vi "Demo.vi"() -> ()   [LabVIEW 2018]
uses:
  Demo_Commands.ctl
panel:
  in  "Scanner brake":bool
  out "new data":bool
  in  "Analog out GAIN":u16(ring) items=["1", "10", "100"]
  in  "Reset":bool
  in  "FIND":bool
  in  "DAF":dbl format="%#_6f"
  out "info string":string="to start measurement press record"
  in  "Scanner Offset":sgl min=-756 max=756
  in  "Scanner Amplitude":sgl=1.0 min=0 max=56
  out "connected":bool=TRUE
  in  "Scanner Frequency":dbl min=0.1 max=25.0
  in  "Sample Frequency":dbl min=0.4 max=50.0
  in  "exit":bool
  in  "Resource":i32(listbox)
  in  "Power Amp":bool
  out "Signalverlaufsgraph":dbl[](graph)
  out "Amplitude":dbl
  in  "Scan":bool
  out "VISA SD":refnum<visa-resource-name>
  out "VISA Error Out":errorcluster
  in  "Connect":bool
  out "ExtTrigFreq (Hz)":dbl format="%.3f"
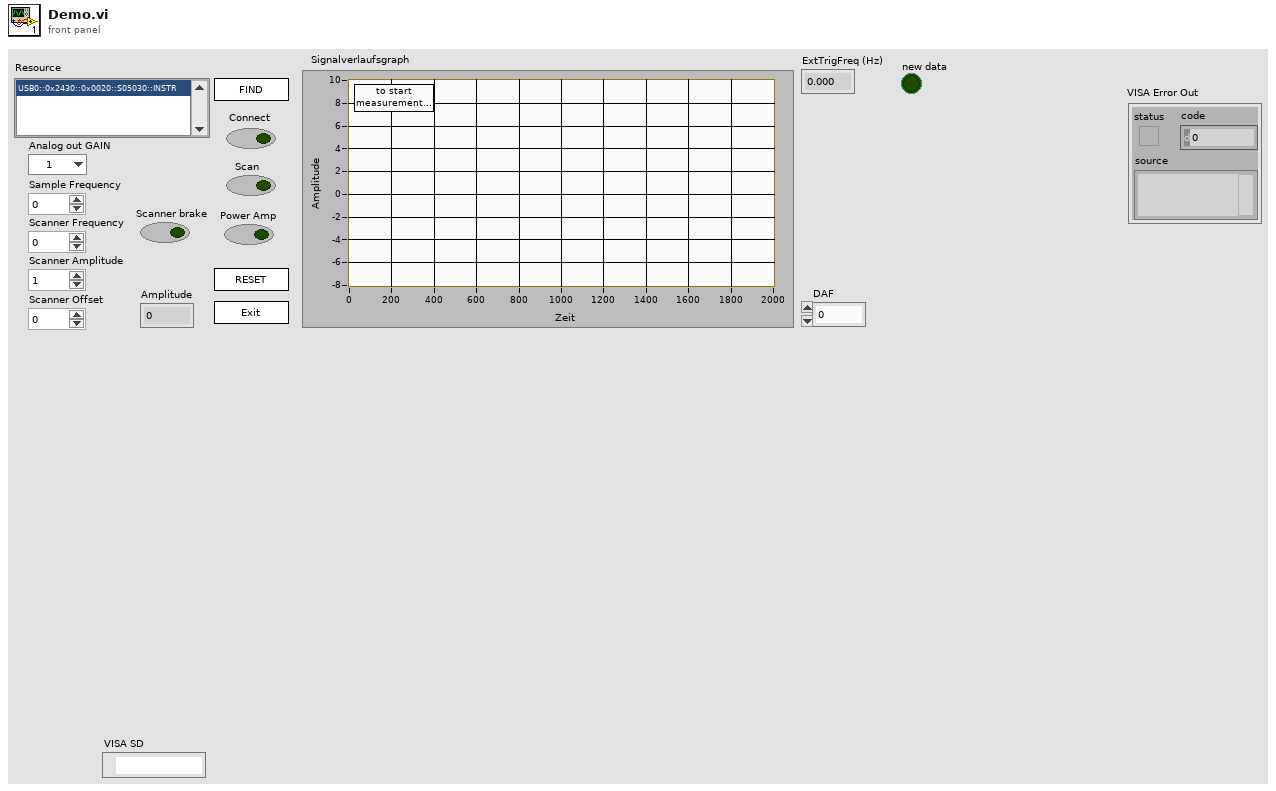
[diagram p1: front panel]
types:
  T1 = typedef "Demo_Commands.ctl" = enum16{"find", "connect", "exit", "get data", "sample frequency", "scan frequency", "power amp", "scanner brake", "reset", "monitor gain", "scan amplitude", "scan offset"}
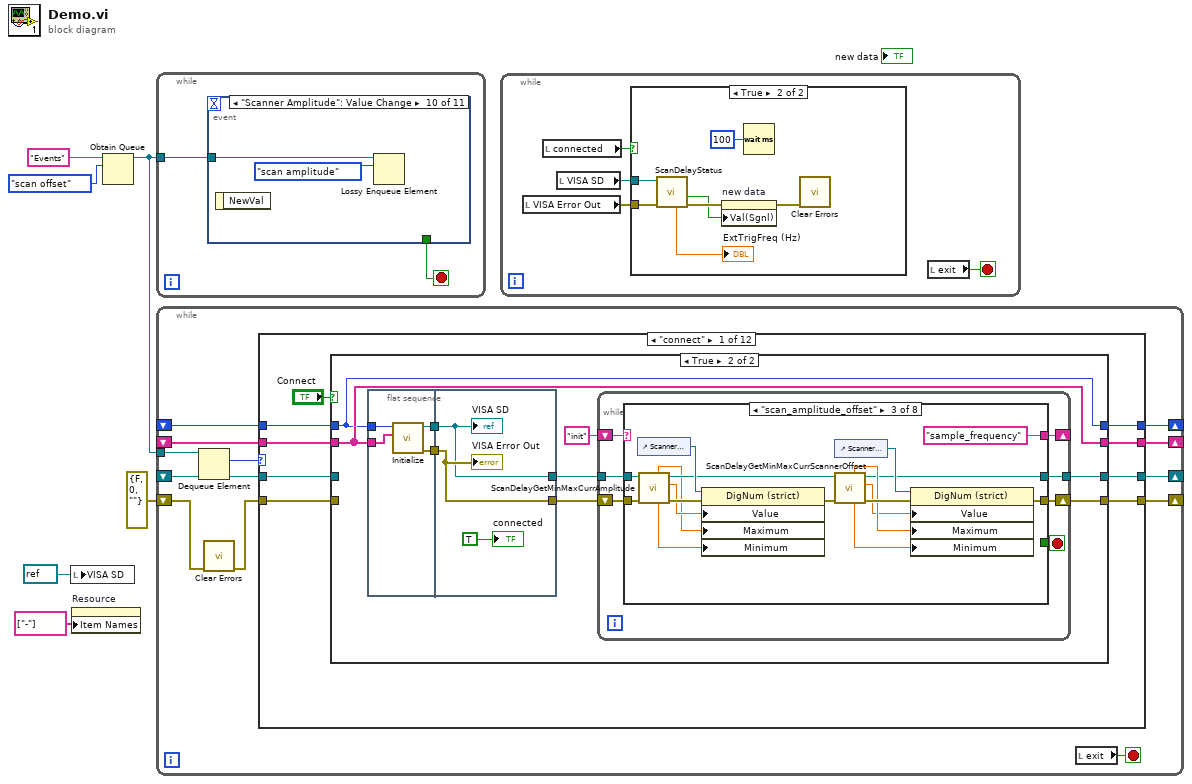
[diagram p0: block diagram]
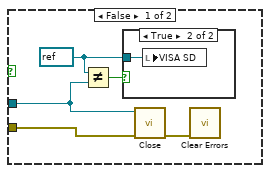
[diagram p2: hidden frame]
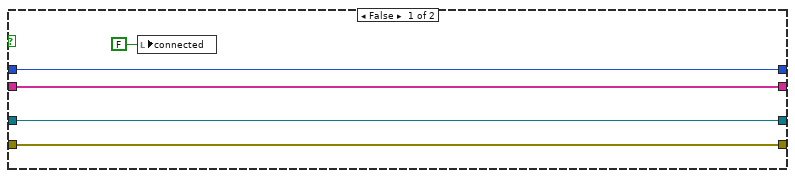
[diagram p4: hidden frame]
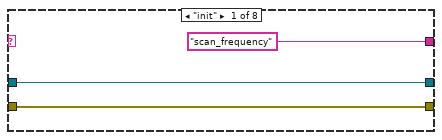
[diagram p5: hidden frame]
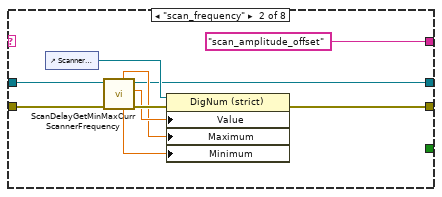
[diagram p6: hidden frame]
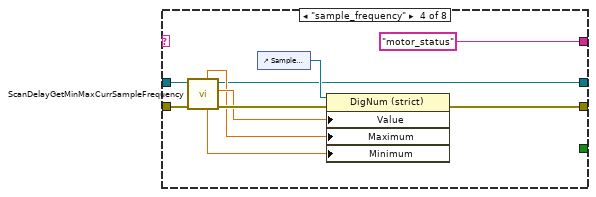
[diagram p7: hidden frame]
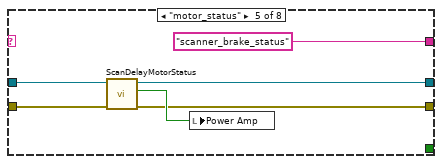
[diagram p8: hidden frame]
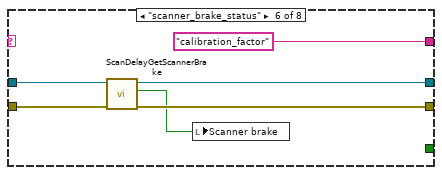
[diagram p9: hidden frame]
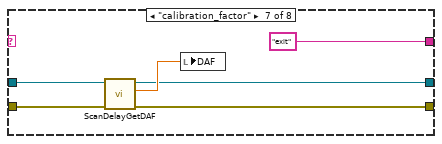
[diagram p10: hidden frame]
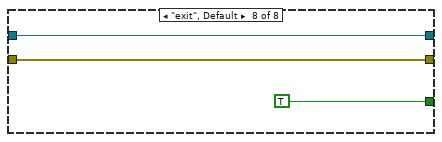
[diagram p11: hidden frame]
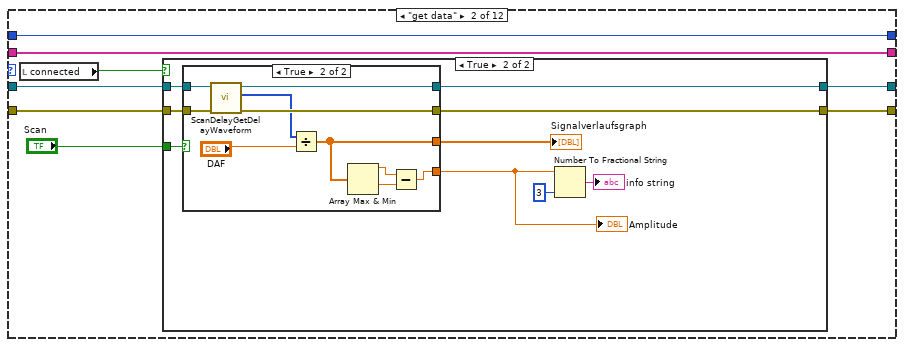
[diagram p12: hidden frame]
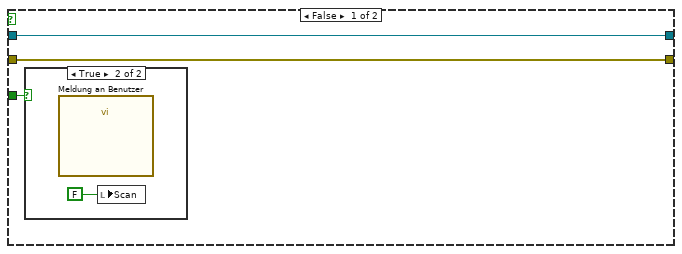
[diagram p13: hidden frame]
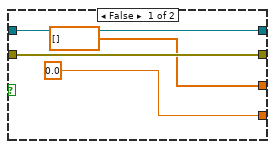
[diagram p15: hidden frame]
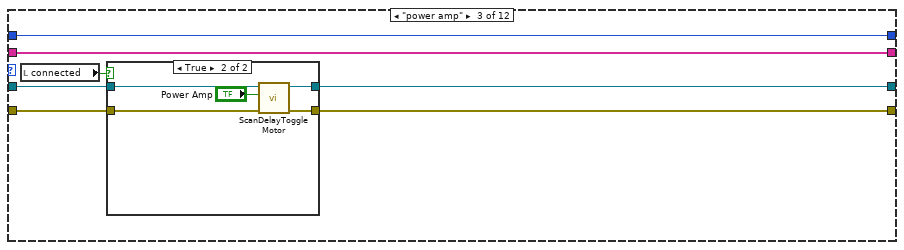
[diagram p16: hidden frame]
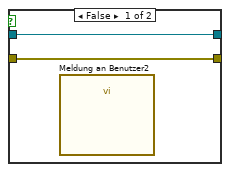
[diagram p17: hidden frame]
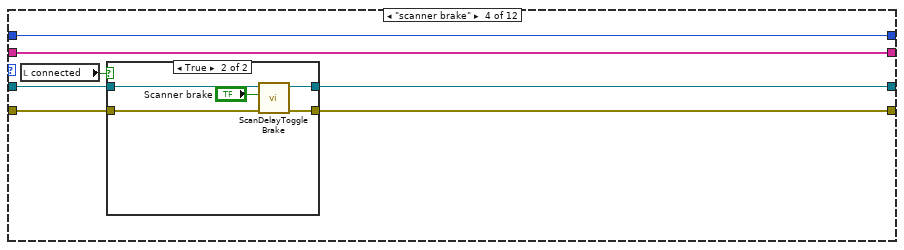
[diagram p18: hidden frame]
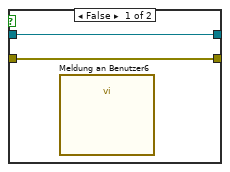
[diagram p19: hidden frame]
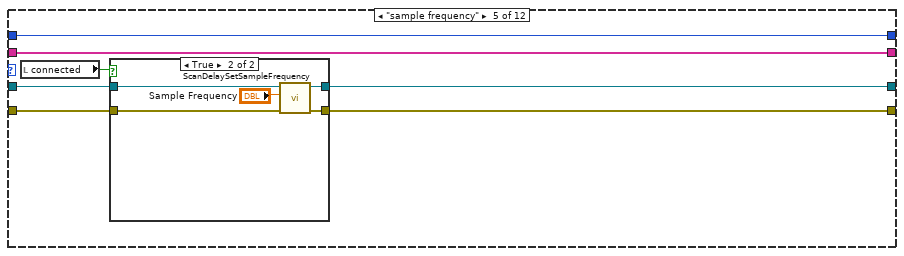
[diagram p20: hidden frame]
diagram:
  n1 = local write "VISA SD"(refnum<visa-resource-name> "0" ("VISA SD")) -> ()
  n2 = property on="Resource" class="LstBox (strict)"("Item Names"=string[] ["-"]) -> ()  [unwired: 2 in, 2 out]
  n3 = Obtain Queue(name (unnamed)="Events" ("Name (unbenannt)"), element data type=Demo_Commands."scan offset" ("element")) -> (queue out=w5:refnum<queue>)  [unwired: 3 in, 2 out]
  n4 = while {
    tunnel: w5 -> [w8]
    stop <- w7 stop-if-true
    n5 = event shown="[9] \"Scanner Amplitude\": Value Change" {
      selector: _ -> [_ _ _ _ _ _ _ _ _ _ _]
      dyn-events: _ -> [_ _ _ _ _ _ _ _ _ _ _]
      timeout: _ -> [_ _ _ _ _ _ _ _ _ _ _]
      tunnel: w8 -> [w10 w12 w15 w17 w19 w21 w23 w25 w27 w29 w31]
      tunnel: [_ _ "exit" _ _ _ _ _ _ _ _] -> w7
      event "FIND": Value Change {
        n6 = event-data() -> ()  [unwired: 1 in, 1 out]
        n7 = Lossy Enqueue Element(queue=w10, element=Demo_Commands."find" ("Befehlssatz")) -> ()  [unwired: 1 in, 4 out]
      }
      event "Connect": Value Change {
        n8 = event-data() -> ()  [unwired: 1 in, 1 out]
        n9 = Lossy Enqueue Element(queue=w12, element=Demo_Commands."connect" ("Befehlssatz")) -> ()  [unwired: 1 in, 4 out]
      }
      event "exit": Value Change {
        n10 = event-data() -> ()  [unwired: 1 in, 1 out]
        n11 = Lossy Enqueue Element(queue=w15, element=Demo_Commands."exit" ("Befehlssatz")) -> ()  [unwired: 1 in, 4 out]
      }
      event "new data", "Scan": Value Change {
        n12 = event-data() -> ()  [unwired: 1 in, 1 out]
        n13 = Lossy Enqueue Element(queue=w17, element=Demo_Commands."get data" ("Befehlssatz")) -> ()  [unwired: 1 in, 4 out]
      }
      event "Reset": Value Change {
        n14 = event-data() -> ()  [unwired: 1 in, 1 out]
        n15 = Lossy Enqueue Element(queue=w19, element=Demo_Commands."reset" ("Befehlssatz")) -> ()  [unwired: 1 in, 4 out]
      }
      event "Sample Frequency": Value Change {
        n16 = event-data() -> ()  [unwired: 1 in, 1 out]
        n17 = Lossy Enqueue Element(queue=w21, element=Demo_Commands."sample frequency" ("Befehlssatz")) -> ()  [unwired: 1 in, 4 out]
      }
      event "Scanner Frequency": Value Change {
        n18 = event-data() -> ()  [unwired: 1 in, 1 out]
        n19 = Lossy Enqueue Element(queue=w23, element=Demo_Commands."scan frequency" ("Befehlssatz")) -> ()  [unwired: 1 in, 4 out]
      }
      event "Analog out GAIN": Value Change {
        n20 = event-data() -> ()  [unwired: 1 in, 1 out]
        n21 = Lossy Enqueue Element(queue=w25, element=Demo_Commands."monitor gain" ("Befehlssatz")) -> ()  [unwired: 1 in, 4 out]
      }
      event "Power Amp": Value Change {
        n22 = event-data() -> ()  [unwired: 1 in, 1 out]
        n23 = Lossy Enqueue Element(queue=w27, element=Demo_Commands."power amp" ("Befehlssatz")) -> ()  [unwired: 1 in, 4 out]
      }
      event "Scanner Amplitude": Value Change {
        n24 = event-data() -> ()  [unwired: 1 in, 1 out]
        n25 = Lossy Enqueue Element(queue=w29, element=Demo_Commands."scan amplitude") -> ()  [unwired: 1 in, 4 out]
      }
      event "Scanner Offset": Value Change {
        n26 = event-data() -> ()  [unwired: 1 in, 1 out]
        n27 = Lossy Enqueue Element(queue=w31, element=Demo_Commands."scan offset") -> ()  [unwired: 1 in, 4 out]
      }
    }
  }
  n28 = while {
    tunnel: w5 -> [w42]
    shift-right: [w41] -> _
    shift-left: _ -> [w36]
    shift-right: [w40] -> _
    shift-left: _ -> [w39]
    shift-right: [w38] -> _
    shift-left: _ -> [w34]
    shift-right: [w37] -> _
    shift-left: errorcluster {"status"=FALSE, "code"=0, "source"=""} ("error out") -> [w33]
    stop <- w35 stop-if-true
    n29 = Dequeue Element(queue=w42) -> (element=w43:T1)  [unwired: 2 in, 3 out]
    n30 = call <vilib>:"Clear Errors.vi"("error in (no error)"=w33) -> ("error out"=w32:errorcluster)  [unwired: 5 in, 1 out]
    n31 = case shown="\"connect\"" w43 {
      tunnel: [w44 w146 w177 w191 w205 w219 w232 "Resource" w243 w260 w275 w289] -> w41
      tunnel: [w45 w147 w178 w192 w206 w220 w235 w239 w244 w259 w274 w288] -> w40
      tunnel: w39 -> [w52 w147 w178 w192 w206 w220 w235 _ w244 w259 w274 w288]
      tunnel: [w50 w148 w180 w194 w208 w222 w233 refnum<visa-resource-name> refnum ("VISA resource name out") w246 w256 w272 w286] -> w38
      tunnel: [w51 w145 w179 w193 w207 w221 w234 w238 w245 w255 w273 w285] -> w37
      tunnel: w36 -> [w49 w146 w177 w191 w205 w219 w232 _ w243 w260 w275 w289]
      tunnel: w34 -> [w47 w144 w181 w195 w209 w223 w233 _ w247 w258 w271 w287]
      tunnel: w32 -> [w46 w143 w182 w196 w210 w224 w234 w236 w248 w257 w270 w284]
      frame "connect" {
        n32 = case shown="True" "Connect" {
          tunnel: w52 -> [w57 w66]
          tunnel: [w53 w62] -> w51
          tunnel: [w54 w61] -> w50
          tunnel: w49 -> [w56 w65]
          tunnel: w47 -> [w54 _]
          tunnel: w46 -> [w53 _]
          tunnel: [w57 w66] -> w45
          tunnel: [w56 w65] -> w44
          frame False {
            n33 = local write "connected"(FALSE ("connected")) -> ()
          }
          frame True {
            n34 = flat-sequence {
              tunnel: w66 -> [w136]
              tunnel: w65 -> [w137]
              tunnel: [w135] -> w59
              tunnel: [w134] -> w58
              tunnel: [w139] -> w63
              tunnel: [w140] -> w64
              tunnel: w59 -> [w140]
              tunnel: w58 -> [w139]
              frame #0 {
                n35 = call "Initialize.vi"("resource array"=w136, "Resource"=w137) -> ("VISA Error Out"=w135:errorcluster, "VISA  name out"=w134:refnum<visa-resource-name>)  [unwired: 7 in, 1 out]
              }
              frame #1 {
                "VISA Error Out" <- w140
                "VISA SD" <- w139
                "connected" <- TRUE
              }
            }
            n36 = while {
              tunnel: w63 -> [w72]
              shift-right: [w71] -> w62
              shift-left: w64 -> [w73]
              tunnel: [w70] -> w61
              shift-right: [w68] -> _
              shift-left: "init" -> [w69]
              stop <- w67 stop-if-true
              n37 = case shown="\"scan_amplitude_offset\"" w69 {
                tunnel: w73 -> [w75 w85 w99 w111 w116 w123 w127 w133]
                tunnel: w72 -> [w74 w84 w98 w110 w115 w122 w126 w132]
                tunnel: [w75 w86 w102 w105 w114 w121 w128 w133] -> w71
                tunnel: [w74 w78 w88 w104 w113 w120 w125 w132] -> w70
                tunnel: ["scan_frequency" "scan_amplitude_offset" "sample_frequency" "motor_status" "scanner_brake_status" "calibration_factor" "exit" _] -> w68
                tunnel: [_ _ _ _ _ _ _ TRUE] -> w67
                frame "init" {
                }
                frame "scan_frequency" {
                  n38 = control-ref of="Scanner Frequency"() -> (w83:refnum<vi>)
                  n39 = call "ScanDelayGetMinMaxCurrScannerFrequency.vi"("error in (no error)"=w85, "VISA resource name in"=w84) -> ("error out"=w82:errorcluster, "value"=w81:dbl, "VISA resource name out"=w78:refnum<visa-resource-name>, "min"=w79:dbl, "max"=w80:dbl)  [unwired: 5 in]
                  n40 = property class="DigNum (strict)"(reference=w83, error in=w82, "Value"=w81, "Maximum"=w80, "Minimum"=w79) -> (error out=w86:errorcluster)  [unwired: 1 out]
                }
                frame "scan_amplitude_offset" {
                  n41 = control-ref of="Scanner Amplitude"() -> (w100:refnum<vi>)
                  n42 = call "ScanDelayGetMinMaxCurrAmplitude.vi"("error in (no error)"=w99, "VISA resource name in"=w98) -> ("error out"=w97:errorcluster, "value"=w95:dbl, "VISA resource name out"=w89:refnum<visa-resource-name>, "min"=w96:dbl, "max"=w87:dbl)  [unwired: 5 in]
                  n43 = property class="DigNum (strict)"(reference=w100, error in=w97, "Value"=w95, "Maximum"=w87, "Minimum"=w96) -> (error out=w102:errorcluster)  [unwired: 1 out]
                  n44 = control-ref of="Scanner Offset"() -> (w90:refnum<vi>)
                  n45 = call "ScanDelayGetMinMaxCurrScannerOffset.vi"("VISA resource name in"=w89) -> ("error out"=w92:errorcluster, "value"=w91:dbl, "VISA resource name out"=w88:refnum<visa-resource-name>, "min"=w94:dbl, "max"=w93:dbl)  [unwired: 6 in]
                  n46 = property class="DigNum (strict)"(reference=w90, error in=w92, "Value"=w91, "Maximum"=w93, "Minimum"=w94) -> ()  [unwired: 2 out]
                }
                frame "sample_frequency" {
                  n47 = call "ScanDelayGetMinMaxCurrSampleFrequency.vi"("error in (no error)"=w111, "VISA resource name in"=w110) -> ("error out"=w109:errorcluster, "value"=w108:dbl, "VISA resource name out"=w104:refnum<visa-resource-name>, "min"=w106:dbl, "max"=w107:dbl)  [unwired: 5 in]
                  n48 = control-ref of="Sample Frequency"() -> (w112:refnum<vi>)
                  n49 = property class="DigNum (strict)"(reference=w112, error in=w109, "Value"=w108, "Maximum"=w107, "Minimum"=w106) -> (error out=w105:errorcluster)  [unwired: 1 out]
                }
                frame "motor_status" {
                  n50 = call "ScanDelayMotorStatus.vi"("error in (no error)"=w116, "VISA resource name in"=w115) -> ("error out"=w114:errorcluster, "value"=w117:bool, "VISA resource name out"=w113:refnum<visa-resource-name>)  [unwired: 7 in]
                  n51 = local write "Power Amp"(w117) -> ()
                }
                frame "scanner_brake_status" {
                  n52 = call "ScanDelayGetScannerBrake.vi"("error in (no error)"=w123, "VISA resource name in"=w122) -> ("error out"=w121:errorcluster, "value"=w119:bool, "VISA resource name out"=w120:refnum<visa-resource-name>)  [unwired: 7 in]
                  n53 = local write "Scanner brake"(w119) -> ()
                }
                frame "calibration_factor" {
                  n54 = call "ScanDelayGetDAF.vi"("error in (no error)"=w127, "VISA resource name in"=w126) -> ("error out"=w128:errorcluster, "value"=w129:dbl, "VISA resource name out"=w125:refnum<visa-resource-name>)  [unwired: 7 in]
                  n55 = local write "DAF"(w129) -> ()
                }
                frame "exit", Default {
                }
              }
            }
          }
        }
      }
      frame "get data" {
        n56 = local read "connected"() -> (w142:bool)
        n57 = case shown="True" w142 {
          tunnel: [w151 w161] -> w148
          tunnel: [w150 w160] -> w145
          tunnel: w144 -> [w151 w159]
          tunnel: w143 -> [w150 w158]
          tunnel: "Scan" -> [w149 w157]
          frame False {
            n58 = case shown="True" w149 {
              frame False {
              }
              frame True {
                n59 = call "Meldung an Benutzer"() -> ()  [unwired: 10 in, 2 out]
                n60 = local write "Scan"(FALSE ("Scann")) -> ()
              }
            }
          }
          frame True {
            n61 = case shown="True" w157 {
              tunnel: w158 -> [w164 w175]
              tunnel: w159 -> [w165 w174]
              tunnel: [w165 w173] -> w161
              tunnel: [w164 w172] -> w160
              tunnel: [dbl[] [] ("PSD Waveform") w169] -> w155
              tunnel: [0.0 ("Amplitude") w166] -> w154
              frame False {
              }
              frame True {
                n62 = call "ScanDelayGetDelayWaveform.vi"("error in (no error)"=w175, "VISA resource name in"=w174) -> ("error out"=w172:errorcluster, "values"=w170:i16[], "VISA resource name out"=w173:refnum<visa-resource-name>)  [unwired: 7 in]
                n63 = Divide(x=w170, y="DAF") -> (x/y=w169:dbl[])
                n64 = Array Max & Min(array=w169) -> (max value=w168:dbl, min value=w167:dbl)  [unwired: 2 out]
                n65 = Subtract(x=w168, y=w167) -> (x-y=w166:dbl)
              }
            }
            "Signalverlaufsgraph" <- w155
            "Amplitude" <- w154
            n66 = Number To Fractional String(number=w154, precision (6)=i16 3) -> (F-format string=→"info string":string)  [unwired: 2 in]
          }
        }
      }
      frame "power amp" {
        n67 = local read "connected"() -> (w176:bool)
        n68 = case shown="True" w176 {
          tunnel: w182 -> [w183 w189]
          tunnel: w181 -> [w184 w188]
          tunnel: [w184 w186] -> w180
          tunnel: [w183 w185] -> w179
          frame False {
            n69 = call "Meldung an Benutzer2"() -> ()  [unwired: 10 in, 2 out]
          }
          frame True {
            n70 = call "ScanDelayToggleMotor.vi"("error in (no error)"=w189, "value"="Power Amp", "VISA resource name in"=w188) -> ("error out"=w185:errorcluster, "VISA resource name out"=w186:refnum<visa-resource-name>)  [unwired: 7 in]
          }
        }
      }
      frame "scanner brake" {
        n71 = local read "connected"() -> (w190:bool)
        n72 = case shown="True" w190 {
          tunnel: w196 -> [w197 w203]
          tunnel: w195 -> [w198 w202]
          tunnel: [w198 w201] -> w194
          tunnel: [w197 w200] -> w193
          frame False {
            n73 = call "Meldung an Benutzer6"() -> ()  [unwired: 10 in, 2 out]
          }
          frame True {
            n74 = call "ScanDelayToggleBrake.vi"("error in (no error)"=w203, "value"="Scanner brake", "VISA resource name in"=w202) -> ("error out"=w200:errorcluster, "VISA resource name out"=w201:refnum<visa-resource-name>)  [unwired: 7 in]
          }
        }
      }
      frame "sample frequency" {
        n75 = local read "connected"() -> (w204:bool)
        n76 = case shown="True" w204 {
          tunnel: w210 -> [w211 w217]
          tunnel: w209 -> [w212 w216]
          tunnel: [w212 w215] -> w208
          tunnel: [w211 w214] -> w207
          frame False {
            n77 = call "Meldung an Benutzer3"() -> ()  [unwired: 10 in, 2 out]
          }
          frame True {
            n78 = call "ScanDelaySetSampleFrequency.vi"("error in (no error)"=w217, "value"="Sample Frequency", "VISA resource name in"=w216) -> ("error out"=w214:errorcluster, "VISA resource name out"=w215:refnum<visa-resource-name>)  [unwired: 7 in]
          }
        }
      }
      frame "scan frequency" {
        n79 = local read "connected"() -> (w218:bool)
        n80 = case shown="True" w218 {
          tunnel: w224 -> [w225 w231]
          tunnel: w223 -> [w226 w230]
          tunnel: [w226 w229] -> w222
          tunnel: [w225 w228] -> w221
          frame False {
            n81 = call "Meldung an Benutzer4"() -> ()  [unwired: 10 in, 2 out]
          }
          frame True {
            n82 = call "ScanDelaySetScannerFrequency.vi"("error in (no error)"=w231, "value"="Scanner Frequency", "VISA resource name in"=w230) -> ("error out"=w228:errorcluster, "VISA resource name out"=w229:refnum<visa-resource-name>)  [unwired: 7 in]
          }
        }
      }
      frame "exit" {
      }
      frame "find" {
        n83 = call "FindResource.vi"("error in (no error)"=w236) -> ("error out"=w238:errorcluster, "resource array"=w241:string[])  [unwired: 8 in, 1 out]
        n84 = property on="Resource" class="LstBox (strict)"("Item Names"=w241) -> ("Item Names"=w239:string[])  [unwired: 2 in, 2 out]
      }
      frame "reset" {
        n85 = local read "connected"() -> (w242:bool)
        n86 = case shown="True" w242 {
          tunnel: w248 -> [w249 w254]
          tunnel: w247 -> [w250 w253]
          tunnel: [w250 w252] -> w246
          tunnel: [w249 w251] -> w245
          frame False {
            n87 = call "Meldung an Benutzer5"() -> ()  [unwired: 10 in, 2 out]
          }
          frame True {
            n88 = call "Reset.vi"("error in (no error)"=w254, "VISA resource name"=w253) -> ("error out"=w251:errorcluster, "VISA resource name out"=w252:refnum<visa-resource-name>)  [unwired: 8 in]
          }
        }
      }
      frame "monitor gain" {
        n89 = local read "connected"() -> (w261:bool)
        n90 = case shown="True" w261 {
          tunnel: w258 -> [w263 w268]
          tunnel: w257 -> [w262 w267]
          tunnel: [w263 w266] -> w256
          tunnel: [w262 w265] -> w255
          frame False {
          }
          frame True {
            n91 = call "ScanDelaySetMonitorGain.vi"("error in (no error)"=w267, "wait"="Analog out GAIN", "VISA resource name in"=w268) -> ("error out"=w265:errorcluster, "VISA resource name out"=w266:refnum<visa-resource-name>)  [unwired: 7 in]
          }
        }
      }
      frame "scan amplitude" {
        n92 = local read "connected"() -> (w269:bool)
        n93 = case shown="True" w269 {
          tunnel: [w276 w282] -> w273
          tunnel: [w277 w281] -> w272
          tunnel: w271 -> [w277 w280]
          tunnel: w270 -> [w276 w279]
          frame False {
          }
          frame True {
            n94 = call "ScanDelaySetAmplitude.vi"("error in (no error)"=w279, "value"="Scanner Amplitude", "VISA resource name in"=w280) -> ("error out"=w282:errorcluster, "VISA resource name out"=w281:refnum<visa-resource-name>)  [unwired: 7 in]
          }
        }
      }
      frame "scan offset" {
        n95 = local read "connected"() -> (w283:bool)
        n96 = case shown="True" w283 {
          tunnel: w287 -> [w291 w296]
          tunnel: [w291 w295] -> w286
          tunnel: [w290 w294] -> w285
          tunnel: w284 -> [w290 w293]
          frame False {
          }
          frame True {
            n97 = call "ScanDelaySetScannerOffset.vi"("error in (no error)"=w293, "value"="Scanner Offset", "VISA resource name in"=w296) -> ("error out"=w294:errorcluster, "VISA resource name out"=w295:refnum<visa-resource-name>)  [unwired: 7 in]
          }
        }
      }
    }
    n98 = local read "exit"() -> (w35:bool)
  }
  n99 = while {
    stop <- w298 stop-if-true
    n100 = local read "VISA Error Out"() -> (w299:errorcluster)
    n101 = local read "connected"() -> (w297:bool)
    n102 = local read "VISA SD"() -> (w300:refnum<visa-resource-name>)
    n103 = case shown="True" w297 {
      tunnel: w300 -> [w303 w313]
      tunnel: w299 -> [w305 w312]
      frame False {
        w302 = refnum<visa-resource-name> "0" ("VISA SD")
        n104 = Not Equal?(x=w302, y=w303) -> (x != y?=w301:bool)
        n105 = case shown="True" w301 {
          tunnel: w302 -> [_ w306]
          frame False {
          }
          frame True {
            n106 = local write "VISA SD"(w306) -> ()
          }
        }
        n107 = call "Close.vi"("error in (no error)"=w305, "VISA resource name"=w303) -> ("error out"=w304:errorcluster)  [unwired: 9 in]
        n108 = call <vilib>:"Clear Errors.vi"("error in (no error)"=w304) -> ()  [unwired: 5 in, 2 out]
      }
      frame True {
        n109 = call "ScanDelayStatus.vi"("error in"=w312, "VISA APE resource"=w313) -> ("error out"=w310:errorcluster, "new data"=w309:bool, "External trigger frequency (Hz)"=→"ExtTrigFreq (Hz)":dbl)  [unwired: 4 in, 3 out]
        n110 = property on="new data" class="Bool (strict)"(error in=w310, "Val(Sgnl)"=w309) -> (error out=w307:errorcluster)  [unwired: 1 in, 1 out]
        n111 = Wait (ms)(milliseconds to wait=u32 100) -> ()  [unwired: 1 out]
        n112 = call <vilib>:"Clear Errors.vi"("error in (no error)"=w307) -> ()  [unwired: 5 in, 2 out]
      }
    }
    n113 = local read "exit"() -> (w298:bool)
  }
